vi "Sea-Level SWI Error Code Interpretor.vi"(1 "Error Code":T1=enum."SEAIO_ERROR_BUSY") -> (0 "error out":errorcluster)   [LabVIEW 2011]
uses:
  TypeDefs/Sea-Level SWI Error Code.ctl
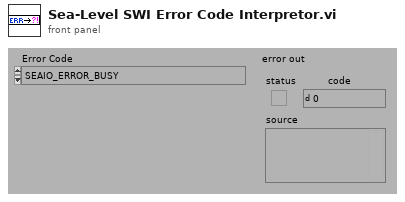
[diagram p1: front panel]
types:
  T1 = typedef "Sea-Level SWI Error Code.ctl" = enum16{"SEAIO_ERROR_NONE", "SEAIO_ERROR_PARAM", "SEAIO_ERROR_NOT_SUPPORTED", "SEAIO_ERROR_PORT_NOT_OPEN", "SEAIO_ERROR_INVALID_NAME", "SEAIO_ERROR_SHARING_VIOLATION", "SEAIO_ERROR_DRIVER_TYPE", "SEAIO_ERROR_BUFFER", "SEAIO_ERROR_INCOMPLETE", "SEAIO_ERROR_GENERAL", "SEAIO_ERROR_IO_PENDING", "SEAIO_ERROR_NO_TXBUFFER", "SEAIO_ERROR_INVALID_DEVICE_REQUEST", "SEAIO_ERROR_INVALID_HANDLE", "SEAIO_ERROR_CANCELED", "SEAIO_ERROR_LAST", "SEAIO_ERROR_NO_MEMORY", "SEAIO_ERROR_BUSY"}
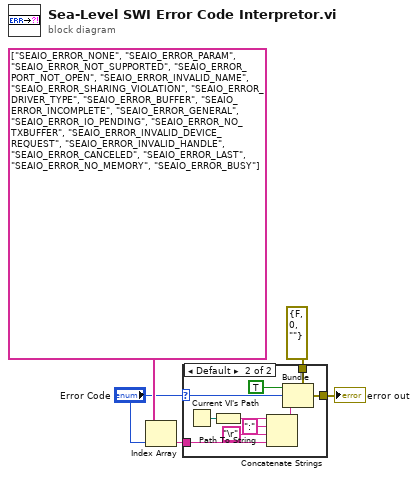
[diagram p0: block diagram]
diagram:
  n1 = Index Array(array=string[] ["SEAIO_ERROR_NONE", "SEAIO_ERROR_PARAM", "SEAIO_ERROR_NOT_SUPPORTED", "SEAIO_ERROR_PORT_NOT_OPEN", "SEAIO_ERROR_INVALID_NAME", "SEAIO_ERROR_SHARING_VIOLATION", "SEAIO_ERROR_DRIVER_TYPE", "SEAIO_ERROR_BUFFER", "SEAIO_ERROR_INCOMPLETE", "SEAIO_ERROR_GENERAL", "SEAIO_ERROR_IO_PENDING", "SEAIO_ERROR_NO_TXBUFFER", "SEAIO_ERROR_INVALID_DEVICE_REQUEST", "SEAIO_ERROR_INVALID_HANDLE", "SEAIO_ERROR_CANCELED", "SEAIO_ERROR_LAST", "SEAIO_ERROR_NO_MEMORY", "SEAIO_ERROR_BUSY"], index="Error Code") -> (element=w2:string)
  n2 = case shown="Default" "Error Code" {
    selector: "Error Code" -> [_ w14]
    tunnel: errorcluster {"status"=FALSE, "code"=0, "source"=""} ("error out") -> [w6 w16]
    tunnel: [w6 w15] -> w3
    tunnel: w2 -> [_ w7]
    frame "SEAIO_ERROR_NONE" {
    }
    frame Default {
      n3 = Current VI's Path() -> (path=w9:path)
      n4 = Path To String(path=w9) -> (string=w10:string)
      n5 = Concatenate Strings(w10, ":" ("string"), "\r", w7) -> (w8:string)
      n6 = Bundle(cluster=w16, "status"=TRUE, "code"=w14, "source"=w8) -> (w15:errorcluster)
    }
  }
  "error out" <- w3
